vi "DMD_Load_Setting.vi"(9 "PixelNum":i32, 10 "DeviceIdPtr":u32, 11 "path in":path) -> (1 "SequenceId":u32, 2 "DeviceId":u32, 3 "path out 2":path, 5 "return type":i32)   [LabVIEW 2016]
panel:
  # "DMD load settings"
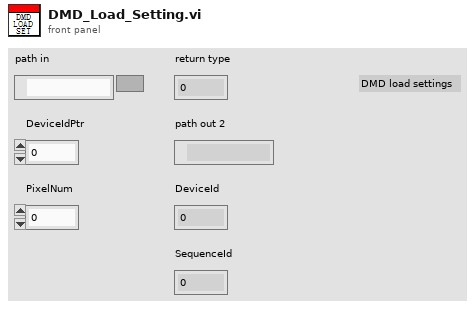
[diagram p1: front panel]
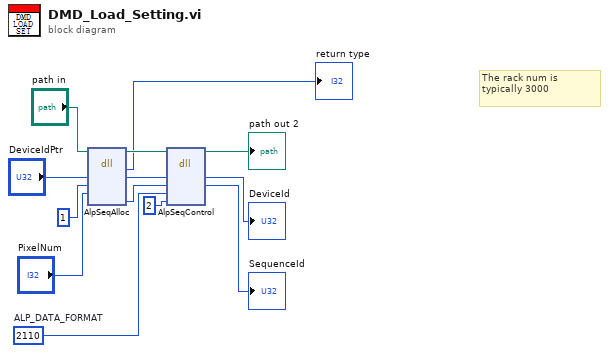
[diagram p0: block diagram]
diagram:
  w1 = 2110  # ALP_DATA_FORMAT
  # "The rack num is typically 3000"
  n1 = dll-call lib="?" fn="AlpSeqAlloc"(path in="path in", "DeviceId"="DeviceIdPtr", "BitPlanes"=1, "PicNum"="PixelNum") -> (path out=w9:path, "return type"=→"return type":i32, "DeviceId"=w7:u32, "SequenceIdPtr"=w10:u32)  [unwired: 5 in, 1 out]
  n2 = dll-call lib="?" fn="AlpSeqControl"(path in=w9, "DeviceId"=w7, "SequenceId"=w10, "ControlType"=w1, "ControlValue"=2) -> (path out=→"path out 2":path, "DeviceId"=→"DeviceId":u32, "SequenceId"=→"SequenceId":u32)  [unwired: 5 in, 1 out]
